vi "DemoSubSubClass1_GOOPKernel.vi"(0 "Ref in":refnum<class "DemoSubSubClass1.lvclass">, 1 "Data in":T6 {"Base class"."Base class"."Attribute1" format="%.2f"}, 2 "Data shared in":T2, 3 "Probe in":string, 6 "Subclass names":string[](array[string]), 7 "error in (no error)":errorcluster, 8 "Action":T5, 9 "Subclass?":bool, 10 "Object name":string, 11 "Class name":string, 13 "Misc":bool, 15 "Occurrence":refnum<k4>, 17 "Occurrence shared":refnum<k4>) -> (14 "Occurrence out":refnum<k4>, 16 "# of objects":i32, 18 "Class\nstatistics":T1, 19 "IsSubclass?":bool, 20 "Ref out":refnum<class "DemoSubSubClass1.lvclass">, 21 "Data out":T6 {"Base class"."Base class"."Attribute1" format="%.2f"}, 22 "Data shared out":T2, 23 "Probe out":string, 25 "Exists?":bool, 26 "Data locked?":bool, 27 "error out":errorcluster)   [LabVIEW 2020, in "DemoSubSubClass1.lvclass"]
doc: "This VIs manages objects of the $CLASS$.\n\n$VERSION$"
uses:
  <vilib>/addons/GOOPUtility/_Demo/GOOPUtil_Demo/DemoSubSubClass1_class/DemoSubSubClass1.lvclass
  <vilib>/addons/GOOPUtility/_Demo/GOOPUtil_Demo/DemoSubSubClass1_class/protected/ObjectAttributes.ctl
  <vilib>/addons/GOOPUtility/_Demo/GOOPUtil_Demo/DemoSubClass1_class/protected/ObjectAttributes.ctl
  <vilib>/addons/GOOPUtility/_Demo/GOOPUtil_Demo/DemoClass1_class/protected/ObjectAttributes.ctl
  <vilib>/addons/_goop3.llb/3GOOPStates.ctl
  C:/Program Files (x86)/National Instruments/LabVIEW 2020/vi.lib/addons/GOOPUtility/_Demo/GOOPUtil_Demo/DemoSubClass1_class/DemoSubClass1.lvclass
  <vilib>/addons/GOOPUtility/_Demo/GOOPUtil_Demo/DemoSubSubClass1_class/protected/ClassAttributes.ctl
  <vilib>/addons/GOOPUtility/_Demo/GOOPUtil_Demo/DemoSubClass1_class/protected/ClassAttributes.ctl
  <vilib>/addons/GOOPUtility/_Demo/GOOPUtil_Demo/DemoClass1_class/protected/ClassAttributes.ctl
  <vilib>/addons/_goop3.llb/3GOOPClassStatistics.ctl
  <vilib>/addons/GOOPUtility/_Demo/GOOPUtil_Demo/DemoSubSubClass1_class/DemoSubSubClass1.lvclass/DemoSubSubClass1.ctl
  <vilib>/addons/GOOPUtility/_Demo/GOOPUtil_Demo/DemoSubClass1_class/DemoSubClass1.lvclass
  <vilib>/addons/GOOPUtility/_Demo/GOOPUtil_Demo/DemoClass1_class/DemoClass1.lvclass
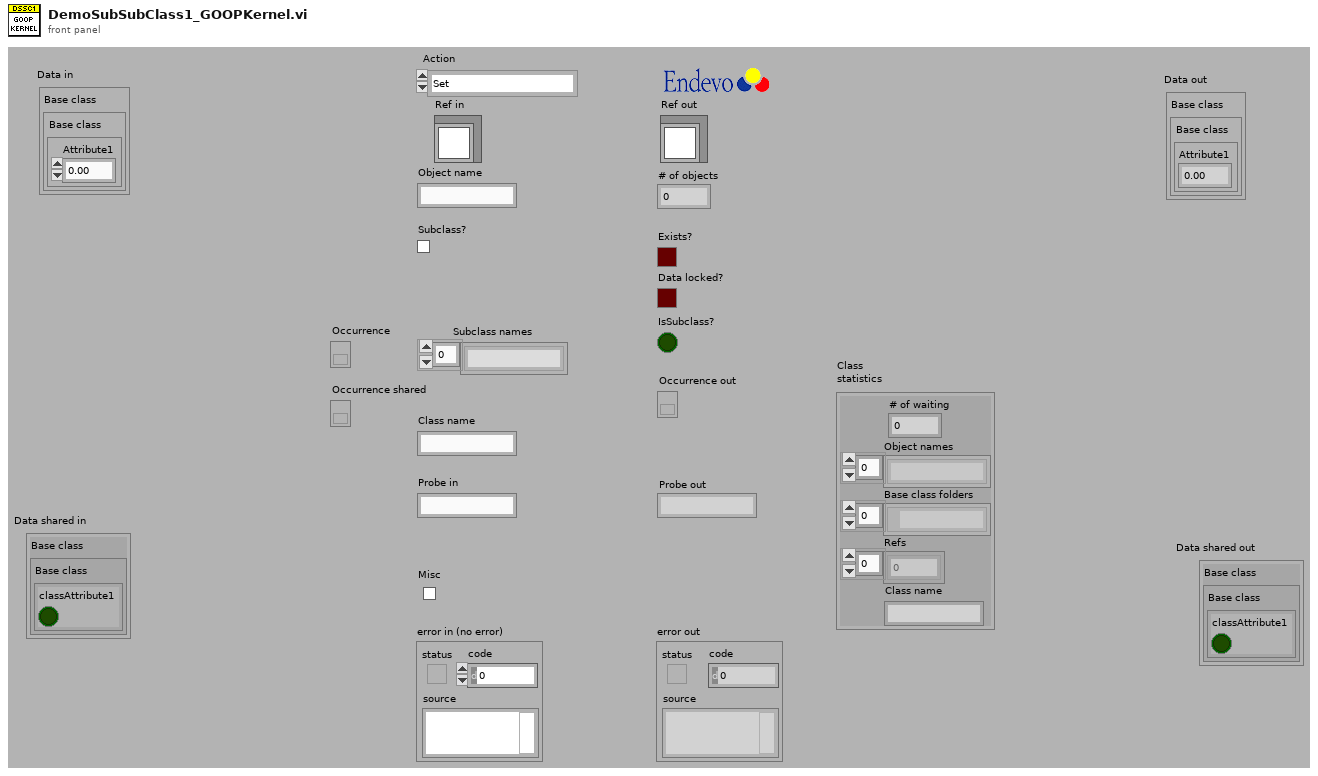
[diagram p1: front panel]
types:
  T1 = typedef "3GOOPClassStatistics.ctl" = cluster{"# of waiting":u32, "Object names":string[], "Base class folders":path[], "Refs":i32[], "Class name":string}
  T2 = typedef "DemoSubSubClass1.lvclass/ClassAttributes.ctl" = cluster{"Base class":T3}
  T3 = typedef "DemoSubClass1.lvclass/ClassAttributes.ctl" = cluster{"Base class":T4}
  T4 = typedef "DemoClass1.lvclass/ClassAttributes.ctl" = cluster{"classAttribute1":bool}
  T5 = typedef "3GOOPStates.ctl" = enum16{"Set", "Get", "New", "Delete", "Clear", "Test and get", "Unlock data", "Information", "Look up existing", "New or look up existing", "Test and get shared", "Get shared", "Set shared", "Unlock shared", "Find dynamic method", "Register dynamic method", "Preload dynamic method", "Probe", "Cast to more generic", "Cast to more specific"}
  T6 = typedef "DemoSubSubClass1.lvclass/ObjectAttributes.ctl" = cluster{"Base class":T7}
  T7 = typedef "DemoSubClass1.lvclass/ObjectAttributes.ctl" = cluster{"Base class":T8}
  T8 = typedef "DemoClass1.lvclass/ObjectAttributes.ctl" = cluster{"Attribute1":dbl}
  T9 = typedef "DemoClass1.lvclass/ObjectReference.ctl" = refnum<k1>
  T10 = cluster{"Name":string, "Subclass":bool, "Class":string}[]
  T11 = cluster{"Name":string, "Subclass":bool, "Class":string}
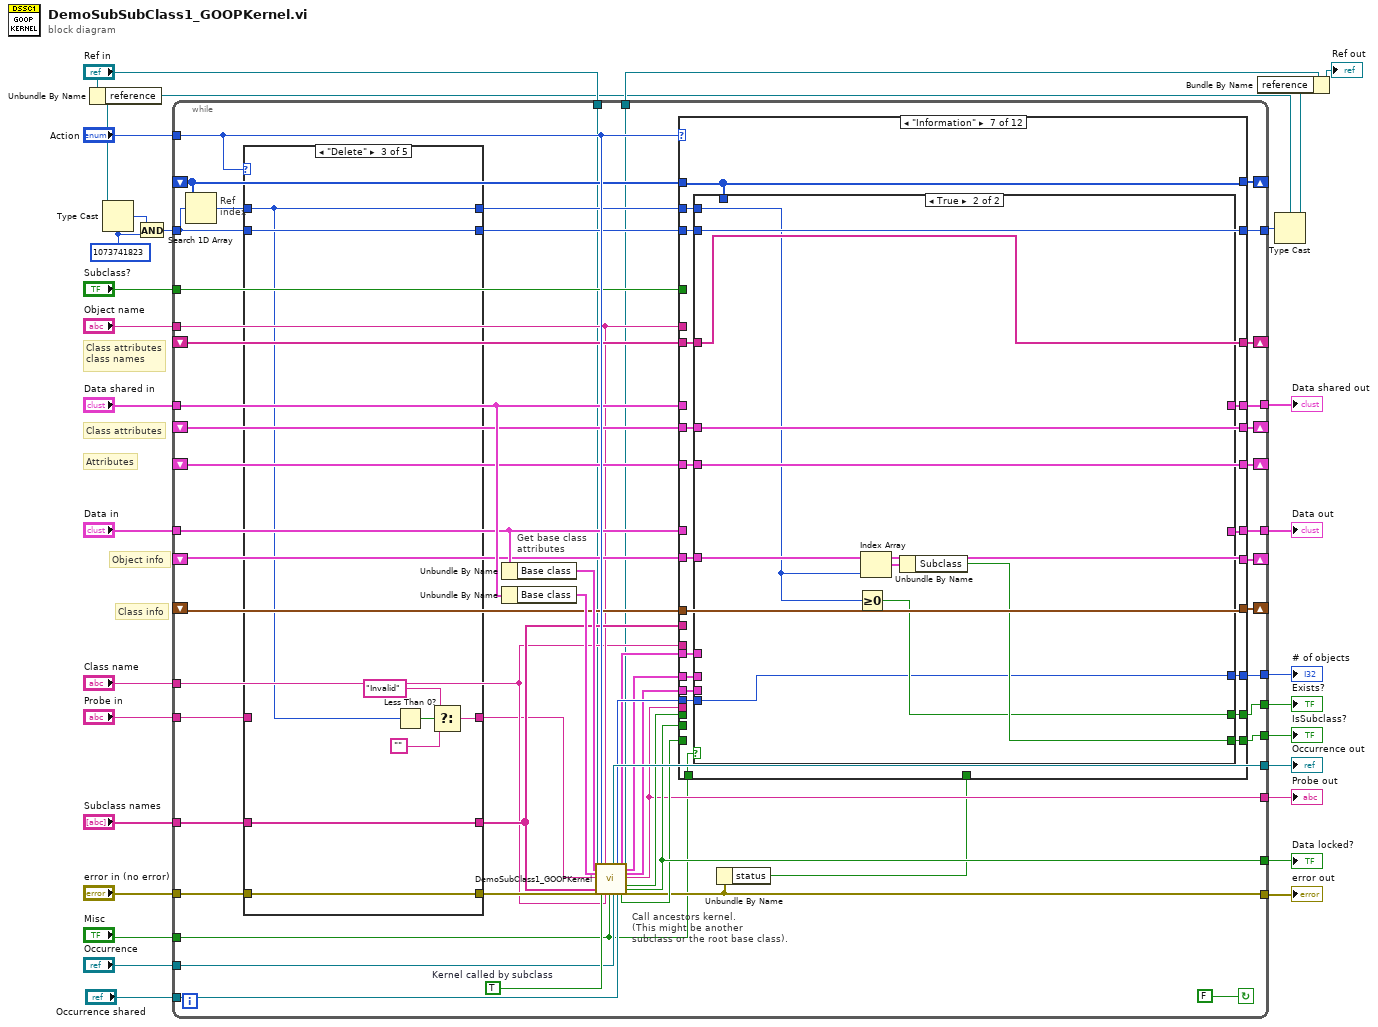
[diagram p0: block diagram]
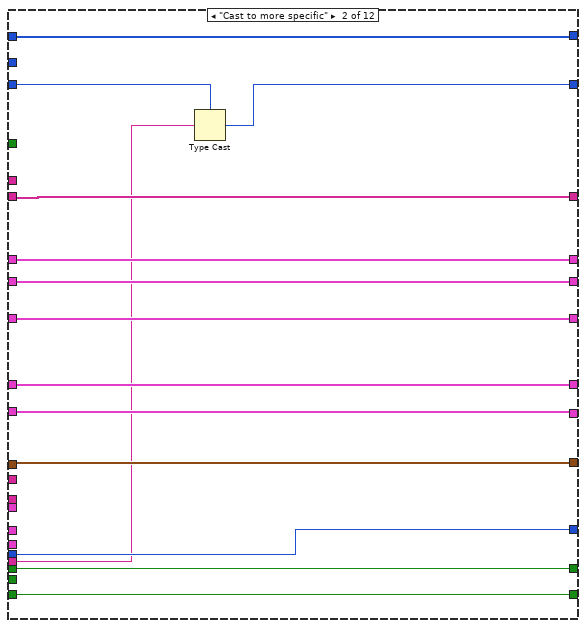
[diagram p3: hidden frame]
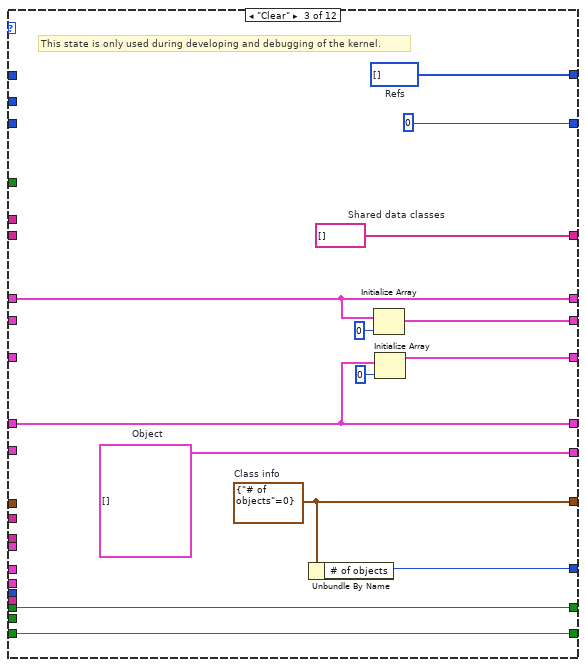
[diagram p4: hidden frame]
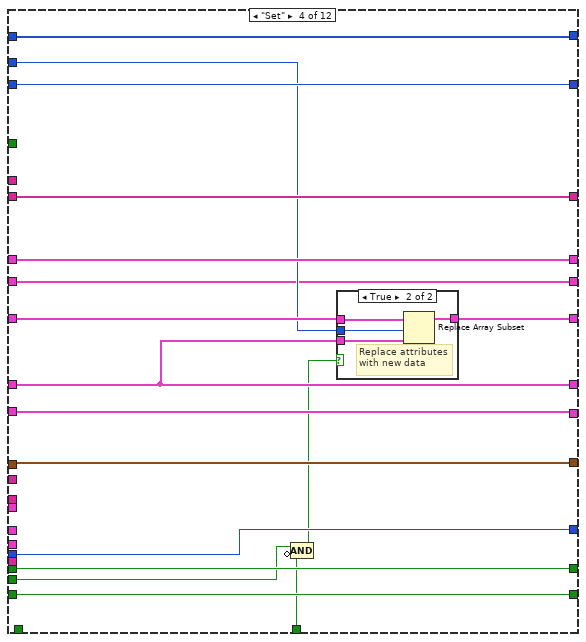
[diagram p5: hidden frame]
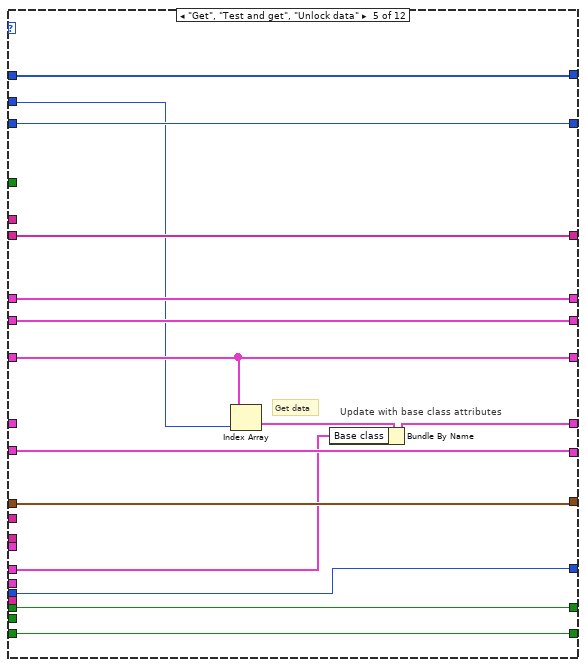
[diagram p7: hidden frame]
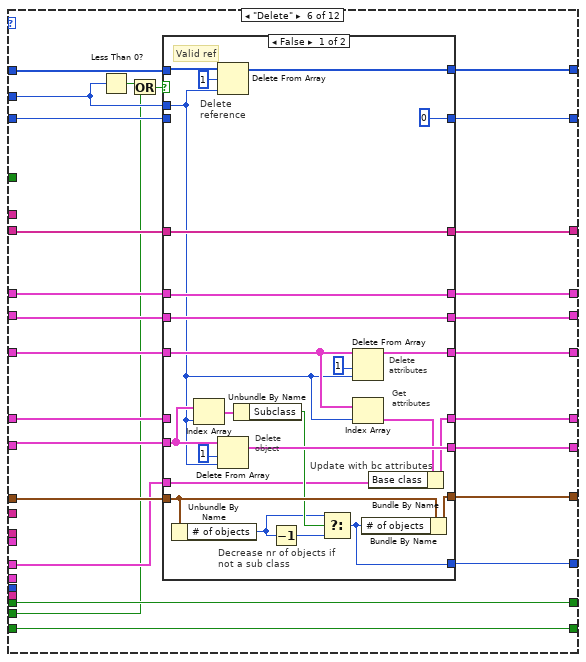
[diagram p8: hidden frame]
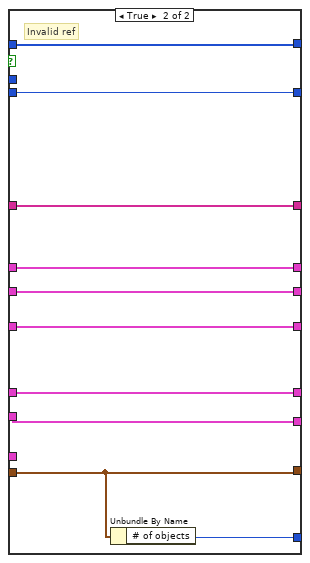
[diagram p9: hidden frame]
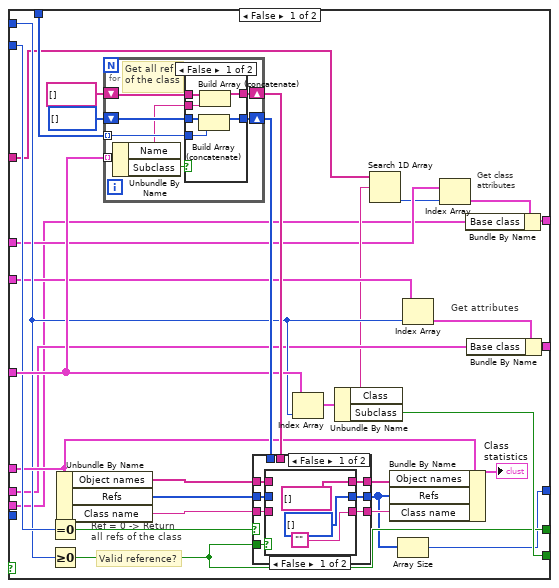
[diagram p10: hidden frame]
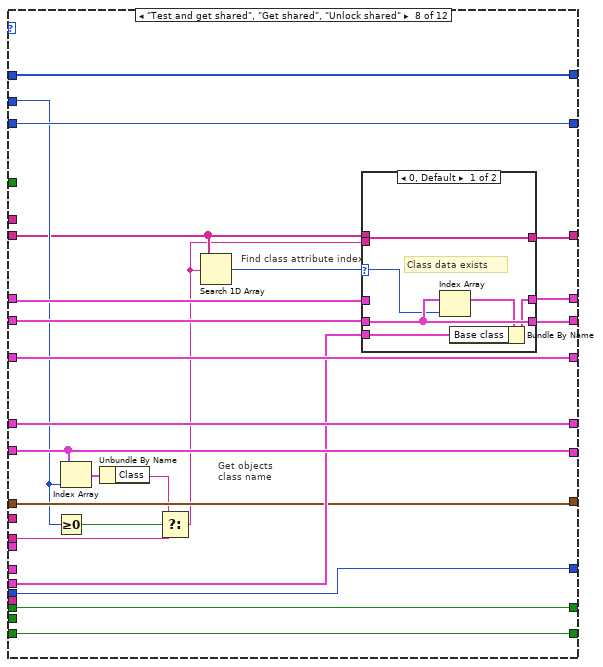
[diagram p14: hidden frame]
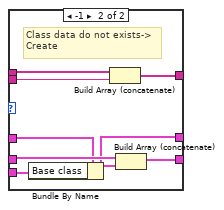
[diagram p15: hidden frame]
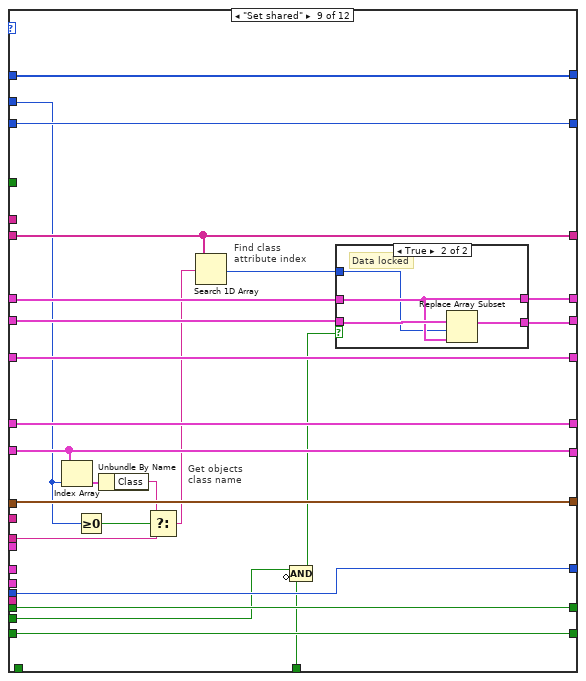
[diagram p16: hidden frame]
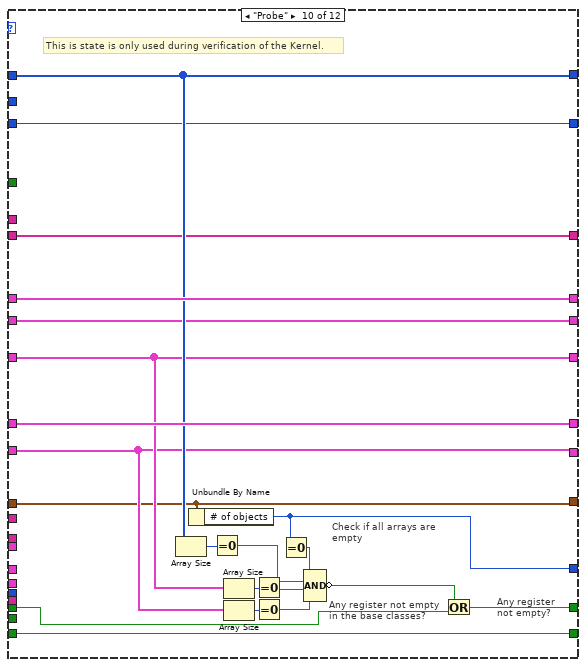
[diagram p18: hidden frame]
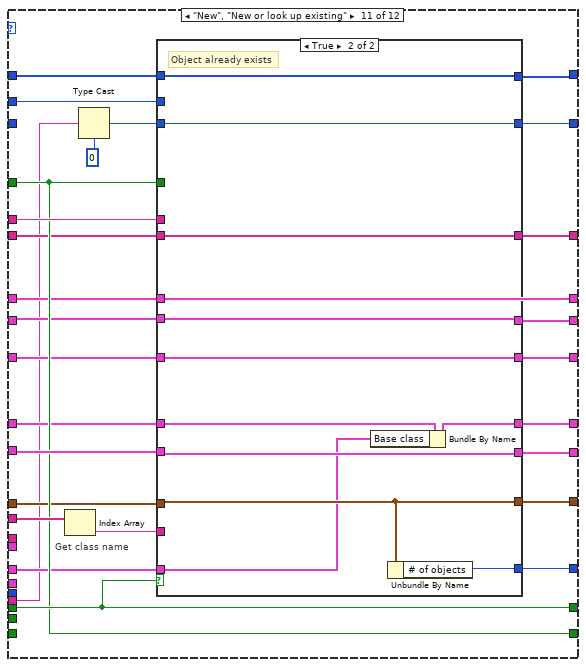
[diagram p19: hidden frame]
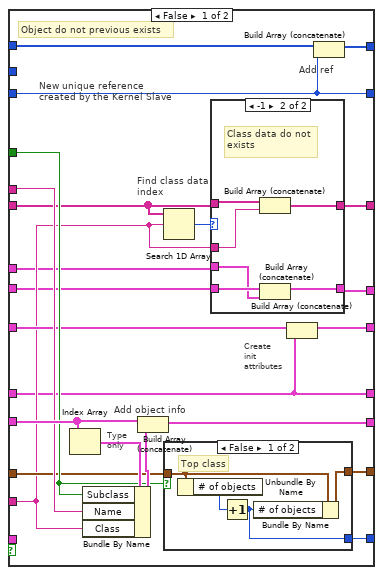
[diagram p20: hidden frame]
diagram:
  w7 = 1073741823 ("x .and. y?")
  # "Class attributes\nclass names"
  # "Attributes"
  # "Class attributes"
  # "Class info"
  # "Object info"
  n1 = Unbundle By Name("Ref in") -> ("reference"=w2:T9)
  n2 = Type Cast(type=w7, x=w2) -> (*(type *) &x=w6:i32)
  n3 = And(x=w6, y=w7) -> (x .and. y?=w11:i32)
  n4 = while {
    tunnel: [w60] -> w13
    tunnel: [w62] -> w14
    tunnel: "Misc" -> [w31]
    shift-left: _ -> [w50]
    shift-right: [w79] -> _
    tunnel: [w69] -> w16
    tunnel: [w46] -> w17
    tunnel: "Subclass names" -> [w71]
    tunnel: "Probe in" -> [w33]
    tunnel: [w40] -> w20
    tunnel: "Class name" -> [w41]
    tunnel: "Data shared in" -> [w76]
    shift-left: _ -> [w64]
    shift-right: [w78] -> _
    shift-left: _ -> [w67]
    shift-right: [w68] -> _
    shift-left: _ -> [w66]
    shift-right: [w65] -> _
    tunnel: [w59] -> w12
    tunnel: "Object name" -> [w42]
    tunnel: [w39] -> w24
    tunnel: "error in (no error)" -> [w80]
    shift-left: _ -> [w52]
    shift-right: [w82] -> _
    tunnel: "Subclass?" -> [w43]
    tunnel: [w49] -> w27
    tunnel: [w81] -> w3
    tunnel: w11 -> [w53]
    shift-left: _ -> [w63]
    shift-right: [w77] -> _
    tunnel: [w70] -> w28
    tunnel: "Action" -> [w83]
    tunnel: "Data in" -> [w73]
    tunnel: "Occurrence" -> [w37]
    tunnel: "Occurrence shared" -> [w36]
    tunnel: [w35] -> w4
    tunnel: "Ref in" -> [w34]
    stop <- FALSE continue-if-true
    w45 = TRUE  # Kernel called by subclass
    # "Call ancestors kernel.\n(This might be another\nsubclass or the root base class)."
    # "Ref\nindex"
    # "Get base class\nattributes"
    n5 = Search 1D Array(1D array=w52, element=w53) -> (index of element=w54:i32)  [unwired: 1 in]
    n6 = case shown="\"Delete\"" w83 {
      tunnel: w80 -> [w493 w500 w508 w515 w528]
      tunnel: [w492 w500 w508 w515 w528] -> w75
      tunnel: w71 -> [w490 w499 w507 w514 w522]
      tunnel: [w490 w499 w507 w514 w523] -> w44
      tunnel: w54 -> [w489 w498 w503 w513 w530]
      tunnel: w53 -> [w491 w497 w506 w511 w529]
      tunnel: [w491 w497 w506 w511 w529] -> w51
      tunnel: [w489 w498 w503 w513 w530] -> w48
      tunnel: w33 -> [w488 w496 _ w509 w519]
      tunnel: [w488 w496 w505 w512 w519] -> w32
      frame "Set", "Get", "Test and get", "Unlock data" {
        # "Check if reference\nis valid"
        n7 = Less Than 0?(x=w489) -> (x < 0?=w494:bool)
        n8 = call <vilib>:"3GOOPSetError.vi"("ref"=w491, "error"=w494, "error in (no error)"=w493, "call depth"=1) -> ("error out"=w492:errorcluster)  [unwired: 15 in]
      }
      frame "Clear", "Information", "Test and get shared".."Probe", Default {
      }
      frame "Delete" {
        n9 = Less Than 0?(x=w503) -> (x < 0?=w504:bool)
        n10 = Select(t="Invalid", s=w504, f="") -> (s? t:f=w505:string)
      }
      frame "Cast to more generic" {
        n11 = Empty String/Path?(string/path=w509) -> (empty?=w510:bool)
        n12 = case shown="False" w510 {
          tunnel: [w516 w518] -> w512
          tunnel: w511 -> [_ w517]
          tunnel: w509 -> [w516 _]
          frame False {
          }
          frame True {
            n13 = Type Cast(x=w517) -> (*(type *) &x=w518:string)  [unwired: 1 in]
          }
        }
      }
      frame "New", "Look up existing", "New or look up existing" {
        # "Find class folder"
        # "Find class name"
        n14 = Current VI's Path() -> (path=w527:path)
        n15 = Strip Path(path=w527) -> (name=w520:string)  [unwired: 1 out]
        n16 = String Length(string=w520) -> (length=w526:i32)
        n17 = Subtract(x=w526, y=13) -> (x-y=w524:i32)
        n18 = String Subset(string=w520, length (rest)=w524) -> (substring=w521:string)  [unwired: 1 in]
        n19 = Build Array (concatenate)(w522, w521) -> (w523:string[])
      }
    }
    n20 = Unbundle By Name(w73) -> ("Base class"=w72:T7)
    n21 = Unbundle By Name(w76) -> ("Base class"=w74:T3)
    n22 = call <vilib>:"DemoSubClass1_GOOPKernel.vi"("Ref in"=w34, "Data in"=w72, "Data shared in"=w74, "Probe in"=w32, "Subclass names"=w44, "error in (no error)"=w75, "Action"=w83, "Subclass?"=w45, "Object name"=w42, "Class name"=w41, "Misc"=w31, "Occurrence"=w37, "Occurrence shared"=w36) -> ("Occurrence out"=w62:refnum<k4>, "# of objects"=w61:i32, "Class\nstatistics"=w58:T1, "IsSubclass?"=w47:bool, "Ref out"=w35:refnum<class "DemoSubSubClass1.lvclass">, "Data out"=w57:T7, "Data shared out"=w56:T3, "Probe out"=w40:string, "Exists?"=w55:bool, "Data locked?"=w49:bool, "error out"=w39:errorcluster)  [unwired: 4 in]
    n23 = Unbundle By Name(w39) -> ("status"=w38:bool)
    n24 = case shown="\"Information\"" w83 {
      tunnel: [w96 w110 w124 w141 w149 w185 w239 w321 w359 w386 w414 w482] -> w82
      tunnel: [w94 w97 0 ("Ref in") w140 w150 w175 w235 w322 w358 w385 w412 w481] -> w81
      tunnel: [w95 w109 w120 w137 w151 w174 w227 w311 w364 w384 w409 w479] -> w79
      tunnel: w76 -> [w93 w108 w116 w136 w153 w184 _ w328 w368 w387 w405 w477]
      tunnel: [w92 w107 w119 w129 w152 w172 w225 w330 w366 w383 w408 w478] -> w78
      tunnel: w73 -> [w90 w105 w117 w130 _ w168 _ w325 w362 w388 w404 w476]
      tunnel: [w91 w106 w118 w139 w159 w181 w230 w326 w363 w382 w411 w480] -> w77
      tunnel: [w90 w105 w117 w130 w157 w169 w229 w325 w362 w388 w402 w474] -> w70
      tunnel: [w93 w108 w116 w136 w153 w183 w226 w329 w369 w387 w405 w477] -> w69
      tunnel: [w88 w103 w113 w134 w161 w177 w237 w318 w360 w379 w416 w484] -> w68
      tunnel: w67 -> [w88 w103 _ w134 w161 w178 w237 w318 w360 w379 w417 w484]
      tunnel: w66 -> [w89 w104 _ w133 w160 w180 w236 w331 w361 w381 w423 w487]
      tunnel: [w89 w104 w115 w133 w160 w179 w236 w331 w361 w381 w422 w487] -> w65
      tunnel: w64 -> [w92 w107 _ w129 w152 w171 w225 w327 w367 w383 w406 w478]
      tunnel: w63 -> [w91 w106 _ w138 w159 w182 w230 w326 w363 w382 w410 w480]
      tunnel: w61 -> [w85 w100 _ w132 w155 _ w222 w319 w357 _ _ _]
      tunnel: [w85 w100 w112 w132 w155 w176 w233 w319 w357 w378 w415 w483] -> w60
      tunnel: [w87 w102 w114 w131 w154 w165 w234 w324 w356 w392 w419 w486] -> w59
      tunnel: w58 -> [_ _ _ _ _ _ w232 _ _ _ _ _]
      tunnel: w57 -> [_ _ _ _ w156 w170 w228 _ _ _ w401 w475]
      tunnel: w56 -> [_ _ _ _ _ _ w224 w320 _ _ _ _]
      tunnel: w55 -> [w87 w102 w114 w131 w154 w165 _ w324 w356 w390 w419 w486]
      tunnel: w52 -> [w96 w110 _ w141 w149 w187 w239 w321 w359 w386 w413 w482]
      tunnel: w51 -> [w94 w98 _ w140 w150 w186 w235 w322 w358 w385 _ _]
      tunnel: w50 -> [w95 w109 _ w137 w151 w173 w227 w313 w364 w384 w407 w479]
      tunnel: w49 -> [_ _ _ w126 _ w162 _ _ w348 _ _ _]
      tunnel: w48 -> [_ _ _ w135 w148 w166 w231 w317 w352 _ w403 _]
      tunnel: w47 -> [w86 w101 w111 w128 w147 w167 _ w323 w355 w389 _ _]
      tunnel: [w86 w101 w111 w128 w147 w167 w238 w323 w355 w389 w418 w485] -> w46
      tunnel: w44 -> [_ _ _ _ _ _ _ _ _ _ w424 _]
      tunnel: w43 -> [_ _ _ _ _ _ _ _ _ _ w418 w485]
      tunnel: w42 -> [_ _ _ _ _ _ _ _ _ _ w420 _]
      tunnel: w41 -> [_ _ _ _ _ _ _ w314 w353 _ _ _]
      tunnel: w40 -> [_ w99 _ _ _ _ _ _ _ _ w398 w473]
      tunnel: w38 -> [_ _ _ w127 _ _ _ _ w349 _ _ _]
      tunnel: w31 -> [_ _ _ _ _ _ w223 _ _ _ _ _]
      frame "Cast to more generic", Default {
      }
      frame "Cast to more specific" {
        n25 = Type Cast(type=w98, x=w99) -> (*(type *) &x=w97:i32)
      }
      frame "Clear" {
        w113 = cluster{"# of objects":i32} {"# of objects"=0}  # Class info
        w115 = T10 []  # Object
        w120 = string[] []  # Shared data classes
        w124 = i32[] []  # Refs
        # "This state is only used during developing and debugging of the kernel."
        n26 = Unbundle By Name(w113) -> ("# of objects"=w112:i32)
        n27 = Initialize Array(w116, 0 ("Dimension Size")) -> (w119:T2[])
        n28 = Initialize Array(w117, 0 ("Dimension Size")) -> (w118:T6[])
      }
      frame "Set" {
        n29 = Compound Arithmetic op=AND(w126, invert w127) -> (w125:bool)
        n30 = case shown="True" w125 {
          tunnel: w130 -> [_ w146]
          tunnel: w138 -> [w142 w145]
          tunnel: [w142 w144] -> w139
          tunnel: w135 -> [_ w143]
          frame False {
            # "Data not locked!"
          }
          frame True {
            # "Replace attributes\nwith new data"
            n31 = Replace Array Subset(array=w145, new element=w146, index=w143) -> (w144:T6[])
          }
        }
      }
      frame "Get", "Test and get", "Unlock data" {
        # "Update with base class attributes"
        # "Get data"
        n32 = Index Array(array=w159, index=w148) -> (element=w158:T6)
        n33 = Bundle By Name(cluster=w158, "Base class"=w156) -> (w157:T6)
      }
      frame "Delete" {
        n34 = Less Than 0?(x=w166) -> (x < 0?=w163:bool)
        n35 = Or(x=w163, y=w162) -> (x .or. y?=w164:bool)
        n36 = case shown="False" w164 {
          tunnel: w187 -> [w210 w219]
          tunnel: w186 -> [_ w218]
          tunnel: [w198 w219] -> w185
          tunnel: w184 -> [w197 w216]
          tunnel: [w197 w216] -> w183
          tunnel: w182 -> [w194 w214]
          tunnel: [w208 w214] -> w181
          tunnel: w180 -> [w205 w213]
          tunnel: [w207 w213] -> w179
          tunnel: w178 -> [w202 w221]
          tunnel: [w203 w221] -> w177
          tunnel: [w200 w220] -> w176
          tunnel: [0 w218] -> w175
          tunnel: [w196 w217] -> w174
          tunnel: w173 -> [w196 w217]
          tunnel: [w195 w215] -> w172
          tunnel: w171 -> [w195 w215]
          tunnel: w170 -> [w191 _]
          tunnel: [w193 w212] -> w169
          tunnel: w168 -> [_ w212]
          tunnel: w166 -> [w190 _]
          frame False {
            # "Update with bc attributes"
            # "Delete\nreference"
            # "Delete\nattributes"
            # "Get\nattributes"
            # "Delete\nobject"
            # "Decrease nr of objects if\nnot a sub class"
            # "Valid ref"
            n37 = Unbundle By Name(w202) -> ("# of objects"=w188:i32)
            n38 = Index Array(array=w205, index=w190) -> (element=w204:T11)
            n39 = Delete From Array(array=w210, length=1 ("Length"), index=w190) -> (array with subset deleted=w198:i32[])  [unwired: 1 out]
            n40 = Delete From Array(array=w205, length=1 ("Length"), index=w190) -> (array with subset deleted=w207:T10)  [unwired: 1 out]
            n41 = Unbundle By Name(w204) -> ("Subclass"=w201:bool)
            n42 = Decrement(x=w188) -> (x-1=w189:i32)
            n43 = Select(t=w188, s=w201, f=w189) -> (s? t:f=w200:i32)
            n44 = Delete From Array(array=w194, length=1 ("Length"), index=w190) -> (array with subset deleted=w208:T6[])  [unwired: 1 out]
            n45 = Index Array(array=w194, index=w190) -> (element=w192:T6)
            n46 = Bundle By Name(cluster=w202, "# of objects"=w200) -> (w203:cluster{"# of objects":i32})
            n47 = Bundle By Name(cluster=w192, "Base class"=w191) -> (w193:T6)
          }
          frame True {
            # "Invalid ref"
            n48 = Unbundle By Name(w221) -> ("# of objects"=w220:i32)
          }
        }
      }
      frame "Information" {
        n49 = case shown="True" w223 {
          tunnel: w239 -> [w269 _]
          tunnel: [w267 w307] -> w238
          tunnel: w236 -> [w259 w309]
          tunnel: w235 -> [w258 _]
          tunnel: [w256 w305] -> w234
          tunnel: [w254 w304] -> w233
          tunnel: w232 -> [w252 _]
          tunnel: w231 -> [w251 w306]
          tunnel: w230 -> [w250 _]
          tunnel: [w249 _] -> w229
          tunnel: w228 -> [w247 _]
          tunnel: w227 -> [w246 _]
          tunnel: [w244 _] -> w226
          tunnel: w225 -> [w243 _]
          tunnel: w224 -> [w240 _]
          tunnel: w222 -> [_ w304]
          frame False {
            # "Valid reference?"
            # "Ref = 0 -> Return\nall refs of the class"
            # "Get class\nattributes"
            # "Get attributes"
            n50 = Equal To 0?(x=w258) -> (x = 0?=w257:bool)
            n51 = Greater Or Equal To 0?(x=w251) -> (x >= 0?=w256:bool)
            n52 = Unbundle By Name(w252) -> ("Object names"=w263:string[], "Refs"=w264:i32[], "Class name"=w265:string)
            n53 = for {
              shift-right: [w294] -> w260
              shift-left: i32[] [] -> [w295]
              tunnel: w269 -> [w293] mode=indexing
              tunnel: w259 -> [w292] mode=indexing
              shift-right: [w289] -> w261
              shift-left: string[] [] ("Object names") -> [w290]
              # "Get all ref\nof the class"
              n54 = Unbundle By Name(w292) -> ("Name"=w288:string, "Subclass"=w291:bool)
              n55 = case shown="False" w291 {
                tunnel: w295 -> [w301 w303]
                tunnel: [w300 w303] -> w294
                tunnel: w293 -> [w299 _]
                tunnel: w290 -> [w298 w302]
                tunnel: [w297 w302] -> w289
                tunnel: w288 -> [w296 _]
                frame False {
                  n56 = Build Array (concatenate)(w301, w299) -> (w300:i32[])
                  n57 = Build Array (concatenate)(w298, w296) -> (w297:string[])
                }
                frame True {
                }
              }
            }
            n58 = case shown="False" w257 {
              tunnel: w256 -> [w278 _]
              tunnel: w264 -> [w277 _]
              tunnel: [w276 w286] -> w255
              tunnel: w265 -> [w275 w285]
              tunnel: [w274 w285] -> w266
              tunnel: w263 -> [w273 _]
              tunnel: [w272 w287] -> w262
              tunnel: w261 -> [_ w287]
              tunnel: w260 -> [_ w286]
              frame False {
                n59 = case shown="False" w278 {
                  tunnel: w277 -> [_ w284]
                  tunnel: [i32[] [] ("Array Constant") w284] -> w276
                  tunnel: w275 -> [_ w283]
                  tunnel: ["" w283] -> w274
                  tunnel: w273 -> [_ w282]
                  tunnel: [string[] [] ("Array Constant") w282] -> w272
                  frame False {
                  }
                  frame True {
                  }
                }
              }
              frame True {
              }
            }
            n60 = Index Array(array=w259, index=w251) -> (element=w268:T11)
            n61 = Unbundle By Name(w268) -> ("Class"=w245:string, "Subclass"=w267:bool)
            n62 = Search 1D Array(1D array=w246, element=w245) -> (index of element=w242:i32)  [unwired: 1 in]
            n63 = Bundle By Name(cluster=w252, "Object names"=w262, "Refs"=w255, "Class name"=w266) -> (→"Class\nstatistics":T1)
            n64 = Array Size(array=w255) -> (size(s)=w254:i32)
            n65 = Index Array(array=w250, index=w251) -> (element=w248:T6)
            n66 = Index Array(array=w243, index=w242) -> (element=w241:T2)
            n67 = Bundle By Name(cluster=w241, "Base class"=w240) -> (w244:T2)
            n68 = Bundle By Name(cluster=w248, "Base class"=w247) -> (w249:T6)
          }
          frame True {
            n69 = Greater Or Equal To 0?(x=w306) -> (x >= 0?=w305:bool)
            n70 = Index Array(array=w309, index=w306) -> (element=w308:T11)
            n71 = Unbundle By Name(w308) -> ("Subclass"=w307:bool)
          }
        }
      }
      frame "Test and get shared", "Get shared", "Unlock shared" {
        # "Find class attribute index"
        # "Get objects\nclass name"
        n72 = Greater Or Equal To 0?(x=w317) -> (x >= 0?=w315:bool)
        n73 = Index Array(array=w331, index=w317) -> (element=w332:T11)
        n74 = Unbundle By Name(w332) -> ("Class"=w316:string)
        n75 = Select(t=w316, s=w315, f=w314) -> (s? t:f=w310:string)
        n76 = Search 1D Array(1D array=w313, element=w310) -> (index of element=w312:i32)  [unwired: 1 in]
        n77 = case shown="0, Default" w312 {
          selector: w312 -> [w333 _]
          tunnel: w327 -> [w338 w346]
          tunnel: [w337 w339] -> w329
          tunnel: [w338 w345] -> w330
          tunnel: w328 -> [_ w344]
          tunnel: w320 -> [w335 w343]
          tunnel: w313 -> [w334 w342]
          tunnel: [w334 w341] -> w311
          tunnel: w310 -> [_ w340]
          frame 0, Default {
            # "Class data exists"
            n78 = Index Array(array=w338, index=w333) -> (element=w336:T2)
            n79 = Bundle By Name(cluster=w336, "Base class"=w335) -> (w337:T2)
          }
          frame -1 {
            # "Class data do not exists->\nCreate"
            n80 = Bundle By Name(cluster=w344, "Base class"=w343) -> (w339:T2)
            n81 = Build Array (concatenate)(w342, w340) -> (w341:string[])
            n82 = Build Array (concatenate)(w346, w339) -> (w345:T2[])
          }
        }
      }
      frame "Set shared" {
        # "Get objects\nclass name"
        # "Find class\nattribute index"
        n83 = Index Array(array=w361, index=w352) -> (element=w370:T11)
        n84 = Greater Or Equal To 0?(x=w352) -> (x >= 0?=w354:bool)
        n85 = Unbundle By Name(w370) -> ("Class"=w351:string)
        n86 = Select(t=w351, s=w354, f=w353) -> (s? t:f=w350:string)
        n87 = Search 1D Array(1D array=w364, element=w350) -> (index of element=w365:i32)  [unwired: 1 in]
        n88 = Compound Arithmetic op=AND(w348, invert w349) -> (w347:bool)
        n89 = case shown="True" w347 {
          tunnel: w368 -> [w372 w374]
          tunnel: w367 -> [w371 w376]
          tunnel: [w371 w375] -> w366
          tunnel: [w372 w374] -> w369
          tunnel: w365 -> [_ w373]
          frame False {
            # "Data not locked"
          }
          frame True {
            # "Data locked"
            n90 = Replace Array Subset(array=w376, new element=w374, index=w373) -> (w375:T2[])
          }
        }
      }
      frame "Probe" {
        # "This is state is only used during verification of the Kernel."
        # "Any register not empty \nin the base classes?"
        # "Any register\nnot empty?"
        # "Check if all arrays are\nempty"
        n91 = Array Size(array=w386) -> (size(s)=w395:i32)
        n92 = Unbundle By Name(w379) -> ("# of objects"=w378:i32)
        n93 = Equal To 0?(x=w395) -> (x = 0?=w380:bool)
        n94 = Array Size(array=w382) -> (size(s)=w397:i32)
        n95 = Array Size(array=w381) -> (size(s)=w396:i32)
        n96 = Equal To 0?(x=w397) -> (x = 0?=w394:bool)
        n97 = Equal To 0?(x=w396) -> (x = 0?=w393:bool)
        n98 = Equal To 0?(x=w378) -> (x = 0?=w377:bool)
        n99 = Compound Arithmetic op=AND(w377, w380, w394, w393) -> (invert w391:bool)
        n100 = Or(x=w391, y=w390) -> (x .or. y?=w392:bool)
      }
      frame "New", "New or look up existing" {
        # "Get class name"
        n101 = Index Array(array=w424) -> (element=w421:string)  [unwired: 1 in]
        n102 = Type Cast(type=0, x=w398) -> (*(type *) &x=w400:i32)
        n103 = case shown="True" w419 {
          tunnel: w423 -> [w444 w468]
          tunnel: [w443 w468] -> w422
          tunnel: w421 -> [w429 _]
          tunnel: w418 -> [w441 _]
          tunnel: w420 -> [w442 _]
          tunnel: w417 -> [w440 w467]
          tunnel: [w439 w467] -> w416
          tunnel: [w438 w466] -> w415
          tunnel: [w437 w471] -> w414
          tunnel: w413 -> [w436 w471]
          tunnel: w400 -> [w435 w464]
          tunnel: [w435 w464] -> w412
          tunnel: [w434 w465] -> w411
          tunnel: w410 -> [w433 w465]
          tunnel: w404 -> [w426 w461]
          tunnel: [w431 w470] -> w409
          tunnel: [w430 w469] -> w408
          tunnel: w407 -> [w425 w470]
          tunnel: w406 -> [w428 w469]
          tunnel: w405 -> [w427 _]
          tunnel: w401 -> [_ w462]
          tunnel: w403 -> [_ _]
          tunnel: [w426 w463] -> w402
          frame False {
            # "Add ref"
            # "Create\ninit\nattributes"
            # "Add object info"
            # "New unique reference\ncreated by the Kernel Slave"
            # "Find class data\nindex"
            # "Object do not previous exists"
            # "Type\nonly"
            n104 = Index Array(array=w444) -> (element=w446:T11)  [unwired: 1 in]
            n105 = Bundle By Name(cluster=w446, "Subclass"=w441, "Name"=w442, "Class"=w429) -> (w445:T11)
            n106 = Build Array (concatenate)(w444, w445) -> (w443:T10)
            n107 = Search 1D Array(1D array=w425, element=w429) -> (index of element=w432:i32)  [unwired: 1 in]
            n108 = case shown="False" w441 {
              tunnel: w440 -> [w458 w460]
              tunnel: [w457 w460] -> w439
              tunnel: [w455 w459] -> w438
              frame False {
                # "Top class"
                n109 = Unbundle By Name(w458) -> ("# of objects"=w456:i32)
                n110 = Increment(x=w456) -> (x+1=w455:i32)
                n111 = Bundle By Name(cluster=w458, "# of objects"=w455) -> (w457:cluster{"# of objects":i32})
              }
              frame True {
                # "Sub class"
                n112 = Unbundle By Name(w460) -> ("# of objects"=w459:i32)
              }
            }
            n113 = case shown="-1" w432 {
              tunnel: w425 -> [w448 w454]
              tunnel: [w448 w453] -> w431
              tunnel: w429 -> [_ w452]
              tunnel: w428 -> [w447 w451]
              tunnel: [w447 w450] -> w430
              tunnel: w427 -> [_ w449]
              frame 0, Default {
                # "Class data already\nexists"
              }
              frame -1 {
                # "Class data do not\nexists"
                n114 = Build Array (concatenate)(w454, w452) -> (w453:string[])
                n115 = Build Array (concatenate)(w451, w449) -> (w450:T2[])
              }
            }
            n116 = Build Array (concatenate)(w433, w426) -> (w434:T6[])
            n117 = Build Array (concatenate)(w436, w435) -> (w437:i32[])
          }
          frame True {
            # "Object already exists"
            n118 = Bundle By Name(cluster=w461, "Base class"=w462) -> (w463:T6)
            n119 = Unbundle By Name(w467) -> ("# of objects"=w466:i32)
          }
        }
      }
      frame "Look up existing" {
        # "Update with base class attributes"
        n120 = Type Cast(type=0, x=w473) -> (*(type *) &x=w481:i32)
        n121 = Bundle By Name(cluster=w476, "Base class"=w475) -> (w474:T6)
        n122 = Unbundle By Name(w484) -> ("# of objects"=w483:i32)
      }
    }
  }
  "Data out" <- w28
  "Data locked?" <- w27
  "error out" <- w24
  "Exists?" <- w12
  "Data shared out" <- w16
  "Probe out" <- w20
  "IsSubclass?" <- w17
  "Occurrence out" <- w14
  "# of objects" <- w13
  n123 = Type Cast(type=w2, x=w3) -> (*(type *) &x=w1:T9)
  n124 = Bundle By Name(cluster=w4, "reference"=w1) -> (→"Ref out":refnum<class "DemoSubSubClass1.lvclass">)
